vi "Operaciones.vi"() -> ()   [LabVIEW 2022 SP3]
panel:
  out "RESIDUO":u8(slide) scale=-1.0..1.0
  out "COCIENTE":dbl(slide) scale=0.0..10.0
  out "PRODUCTO":dbl(knob) scale=0.0..10.0
  out "NÚMERO":bool
  out "NÚMERO":bool
  out "EJERCICIO 4":dbl
  out "REDONDEO":dbl
  out "RESULTADO":dbl
  out "RESULTADO":dbl
  out "RESULTADO":dbl
  in  "NÚMERO B":dbl
  in  "NÚMERO A":dbl
  # "EJERCICIO 1"
  # "EJERCICIO 2"
  # "BLANCO -> NÚMERO POSITIVO"
  # "NEGRO -> NÚMERO NEGATIVO"
  # "EJERCICIO 3"
  # "EJERCICIO 4"
  # "BLANCO -> NÚMERO POSITIVO"
  # "NEGRO -> NÚMERO NEGATIVO"
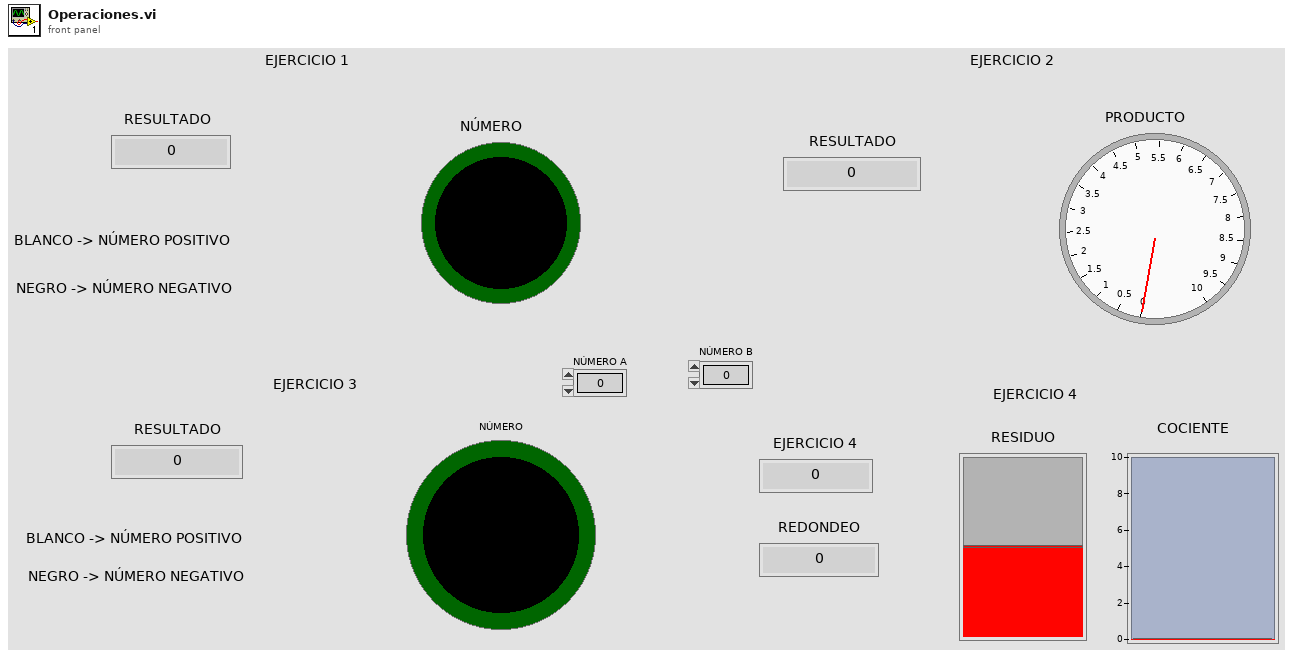
[diagram p1: front panel]
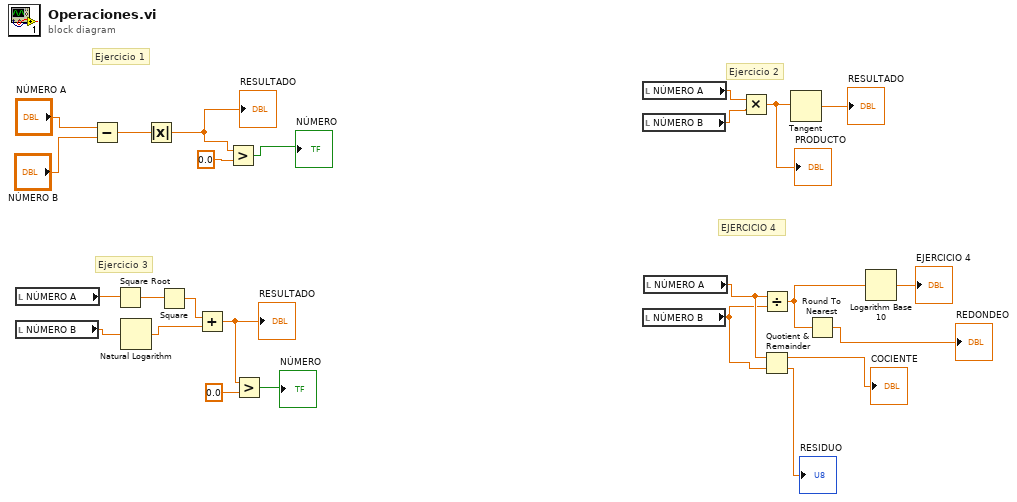
[diagram p0: block diagram]
diagram:
  # "EJERCICIO 4"
  # "Ejercicio 3"
  # "Ejercicio 2"
  # "Ejercicio 1"
  n1 = local read "NÚMERO A"() -> (w23:dbl)
  n2 = local read "NÚMERO B"() -> (w21:dbl)
  n3 = Subtract(x="NÚMERO A", y="NÚMERO B") -> (x-y=w15:dbl)
  n4 = Square Root(x=w23) -> (sqrt(x)=w22:dbl)
  n5 = Natural Logarithm(1:w21) -> (0:w19:dbl)
  n6 = Absolute Value(x=w15) -> (abs(x)=w12:dbl)
  "RESULTADO" <- w12
  n7 = Square(x=w22) -> (x^2=w20:dbl)
  n8 = Add(x=w20, y=w19) -> (x+y=w10:dbl)
  "RESULTADO" <- w10
  n9 = Greater?(x=w12, y=0.0) -> (0:→"NÚMERO":bool)
  n10 = Greater?(x=w10, y=0.0) -> (0:→"NÚMERO":bool)
  n11 = local read "NÚMERO A"() -> (w8:dbl)
  n12 = local read "NÚMERO B"() -> (w7:dbl)
  n13 = local read "NÚMERO B"() -> (w3:dbl)
  n14 = local read "NÚMERO A"() -> (w4:dbl)
  n15 = Multiply(x=w8, y=w7) -> (x*y=w6:dbl)
  "PRODUCTO" <- w6
  n16 = Divide(x=w4, y=w3) -> (x/y=w5:dbl)
  n17 = Quotient & Remainder(x=w4, y=w3) -> (x-y*floor(x/y)=→"COCIENTE":dbl, floor(x/y)=→"RESIDUO":dbl)
  n18 = Tangent(1:w6) -> (0:→"RESULTADO":dbl)
  n19 = Round To Nearest(number=w5) -> (nearest integer value=→"REDONDEO":dbl)
  n20 = Logarithm Base 10(1:w5) -> (0:→"EJERCICIO 4":dbl)
